vi "Init_Test.vi"(8 "error in (no error)":errorcluster caption="entrée d'erreur (pas d'erreur)", 11 "Get_Voltage en entrée":refnum<class "Enable_Relay.lvclass">) -> (0 "error out":errorcluster caption="sortie d'erreur", 3 "Get_Voltage en sortie":refnum<class "Enable_Relay.lvclass">)   [LabVIEW 2020, in "Library Test.lvlib" / "Enable_Relay.lvclass"]
uses:
  Enable_Relay.lvclass
  C:/Users/ngarcin/OneDrive - Altyor/Standard TB/Class/Test/Test (Default)/Test (Default).lvclass
  Commun VI/TypeDef/Commande Test/Commande Value Type.ctl
  Commun VI/TypeDef/Commande Test/Commande Type Test.ctl
  Commun VI/TypeDef/Commande Relay_Board/Data_Write_Relay_Board.ctl
  Commun VI/TypeDef/Commande Relay_Board/Parameter Relay_Board.ctl
  Relay_Board/Relay_Board (Default)/Class Relay_Board (Default).lvclass
  JSON API/JSON Value/Set from JSON string.vi
  JSON API/Variant JSON/Variant to JSON.vi
  JSON API/JSON Value/Get Item by name array.vi
  Test_Wtih_Instr/Test_With_Inst.lvclass
  Instrument/Instrument (Default)/Class Instrument (Default).lvclass
  JSON API/JSON Value/JSON Value.lvclass
  Enable_Relay.lvclass/Enable_Relay.ctl
  Commun VI/Library Commun.lvlib
  JSON API/Get Polymorphic/JSON GetSet.lvlib
  JSON API/Variant JSON/Variant JSON.lvlib
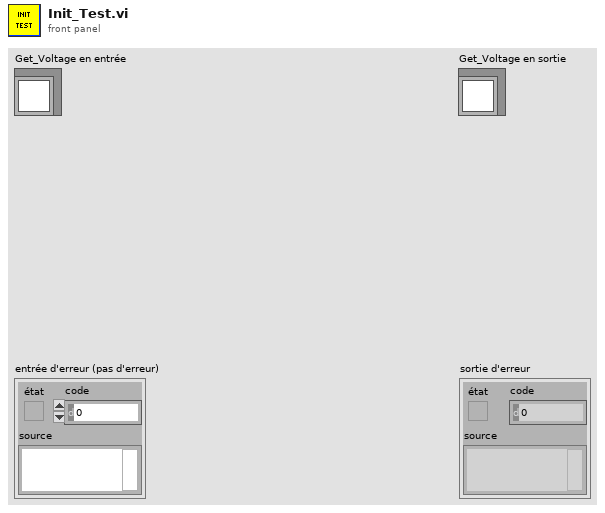
[diagram p1: front panel]
types:
  T1 = typedef "Library Commun.lvlib/Commande Type Test.ctl" = enum16{"Function", "Test", "Calculation"}
  T2 = typedef "Library Commun.lvlib/Commande Value Type.ctl" = enum16{"None", "String", "Number", "Timestamp", "Boolean", "Array"}
  T3 = typedef "Library Commun.lvlib/Data_Write_Relay_Board.ctl" = enum16{"Enable Relays", "Disable Relays"}
  T4 = typedef "Library Commun.lvlib/Parameter Relay_Board.ctl" = cluster{"Device_Com_Port":string, "Address Board":string, "Tab_Num_Relay":u8[], "Parameter Class Relay_Board":refnum<class "Class Relay_Board (Default).lvclass">}
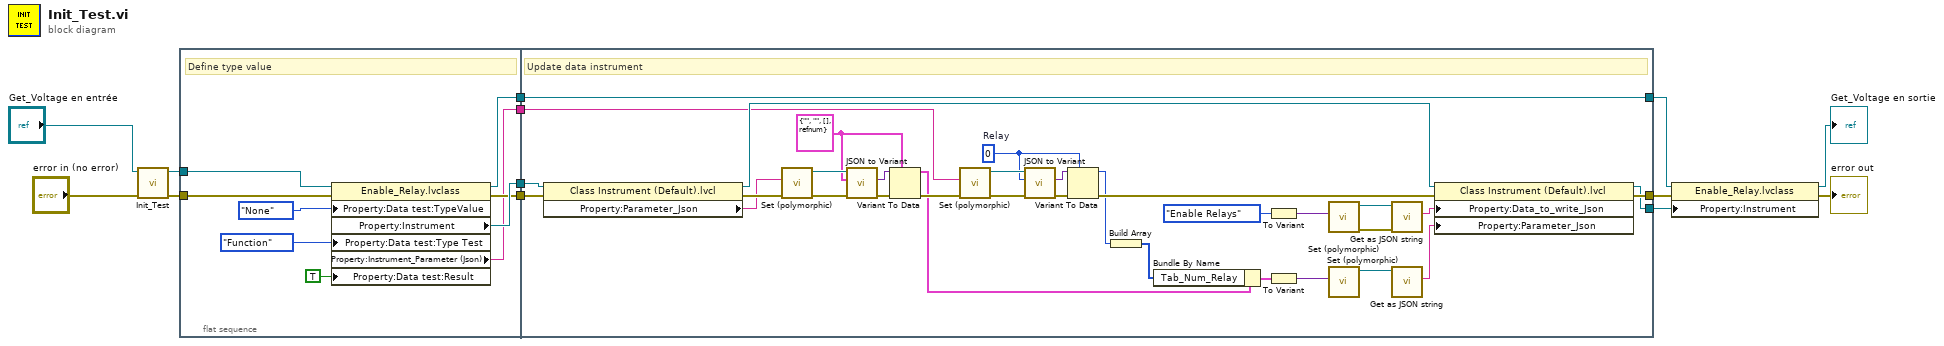
[diagram p0: block diagram]
diagram:
  n1 = call-parent "Init_Test.vi"("error in (no error)"="error in (no error)", "Test_With_Inst en entrée"="Get_Voltage en entrée") -> ("error out"=w10:errorcluster, "Test_With_Inst en sortie"=w11:refnum<class "Enable_Relay.lvclass">)  [unwired: 8 in]
  n2 = flat-sequence {
    tunnel: w11 -> [w22]
    tunnel: w10 -> [w21]
    tunnel: [w20] -> w9
    tunnel: [w19] -> w3
    tunnel: [w16] -> w2
    tunnel: [w15] -> w1
    tunnel: [w55] -> w6
    tunnel: [w54] -> w7
    tunnel: w9 -> [w53]
    tunnel: [w53] -> w8
    tunnel: w3 -> [w47]
    tunnel: w2 -> [w45]
    tunnel: w1 -> [w40]
    frame #0 {
      # "Define type value"
      n3 = property class="Enable_Relay.lvclass"(reference=w22, error in=w21, "Property:Data test:TypeValue"=Commande_Value_Type."None" ("TypeValue"), "Property:Data test:Type Test"=Commande_Type_Test."Function" ("Type Test"), "Property:Data test:Result"=TRUE ("Result")) -> (reference out=w20:refnum<class "Enable_Relay.lvclass">, error out=w16:errorcluster, "Property:Instrument"=w19:refnum<class "Class Instrument (Default).lvclass">, "Property:Instrument_Parameter (Json)"=w15:string)
    }
    frame #1 {
      w31 = T4 {"Device_Com_Port"="", "Address Board"="", "Tab_Num_Relay"=[], "Parameter Class Relay_Board"=refnum} ("Parameter")
      w30 = 0  # Relay
      # "Update data instrument"
      n4 = property class="Class Instrument (Default).lvcl"(reference=w47, error in=w45) -> (reference out=w46:refnum<class "Class Instrument (Default).lvclass">, error out=w34:errorcluster, "Property:Parameter_Json"=w23:string)
      n5 = call-poly "Set (polymorphic).vi"("error in (no error)"=w34, "JSON stream"=w23) -> ("error out"=w37:errorcluster, "JSON Value out"=w39:refnum<class "JSON Value.lvclass">)  [unwired: 7 in, 1 out]
      n6 = call "JSON to Variant.vi"("error in (no error)"=w37, "Variant (Data Type)"=w31, "JSON Value"=w39) -> ("error out"=w38:errorcluster, "Variant out"=w36:variant)  [unwired: 7 in]
      n7 = Variant To Data(error in=w38, type=w31, Variant=w36) -> (data=w32:T4, error out=w35:errorcluster)
      n8 = call-poly "Set (polymorphic).vi"("error in (no error)"=w35, "JSON stream"=w40) -> ("error out"=w43:errorcluster, "JSON Value out"=w41:refnum<class "JSON Value.lvclass">)  [unwired: 7 in, 1 out]
      n9 = call "JSON to Variant.vi"("error in (no error)"=w43, "Variant (Data Type)"=w30, "JSON Value"=w41) -> ("error out"=w42:errorcluster, "Variant out"=w44:variant)  [unwired: 7 in]
      n10 = Variant To Data(error in=w42, type=w30, Variant=w44) -> (data=w24:i32, error out=w33:errorcluster)
      n11 = Build Array(w24) -> (w29:i32[])
      n12 = Bundle By Name(cluster=w32, "Tab_Num_Relay"=w29) -> (w27:T4)
      n13 = To Variant(anything=Data_Write_Relay_Board."Enable Relays" ("Function")) -> (Variant=w52:variant)
      n14 = To Variant(anything=w27) -> (Variant=w26:variant)
      n15 = call-poly "Set (polymorphic).vi"("Variant"=w52) -> ("error out"=w50:errorcluster, "JSON Value out"=w51:refnum<class "JSON Value.lvclass">)  [unwired: 9 in]
      n16 = call-poly "Set (polymorphic).vi"("Variant"=w26) -> ("JSON Value out"=w28:refnum<class "JSON Value.lvclass">)  [unwired: 9 in, 1 out]
      n17 = call "Get as JSON string.vi"("error in (no error)"=w50, "JSON Value in"=w51) -> ("<JSON>"=w49:string)  [unwired: 8 in, 1 out]
      n18 = call "Get as JSON string.vi"("JSON Value in"=w28) -> ("<JSON>"=w25:string)  [unwired: 9 in, 1 out]
      n19 = property class="Class Instrument (Default).lvcl"(reference=w46, error in=w33, "Property:Data_to_write_Json"=w49, "Property:Parameter_Json"=w25) -> (reference out=w54:refnum<class "Class Instrument (Default).lvclass">, error out=w55:errorcluster)
    }
  }
  n20 = property class="Enable_Relay.lvclass"(reference=w8, error in=w6, "Property:Instrument"=w7) -> (reference out=→"Get_Voltage en sortie":refnum<class "Enable_Relay.lvclass">, error out=→"error out":errorcluster)
